vi "Create Threshold Event.vi"(0 "Threshold control":bool, 1 "Release dur. (ms)":u32, 2 "Scenario dur. (ms)":u32, 3 "Precheck dur. (ms)":u32, 5 "Threshold value":dbl, 7 "Threshold reached":bool, 9 "queue":refnum<queue>, 11 "error in":errorcluster, 13 "Queue is empty":bool) -> (15 "error out":errorcluster)   [LabVIEW 2024]
uses:
  Type Definitions/Threshold Event Parameters.ctl
  Type Definitions/Threshold Events.ctl
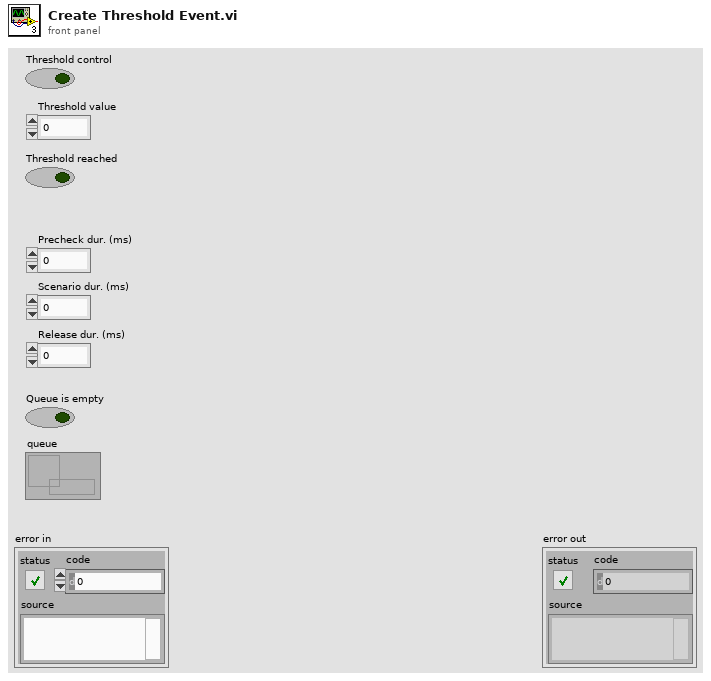
[diagram p1: front panel]
types:
  T1 = typedef "Threshold Events.ctl" = enum16{"Start Precheck", "Start Scenario", "Start Releasing", "Finish Releasing", "Clear Scenario", "Abort Scenario"}
  T2 = typedef "Threshold Event Parameters.ctl" = cluster{"Event Start time":u32, "Event name":T1, "Threshold value":dbl, "Precheck duration":u32, "Scenario Duration":u32, "Release duration":u32}
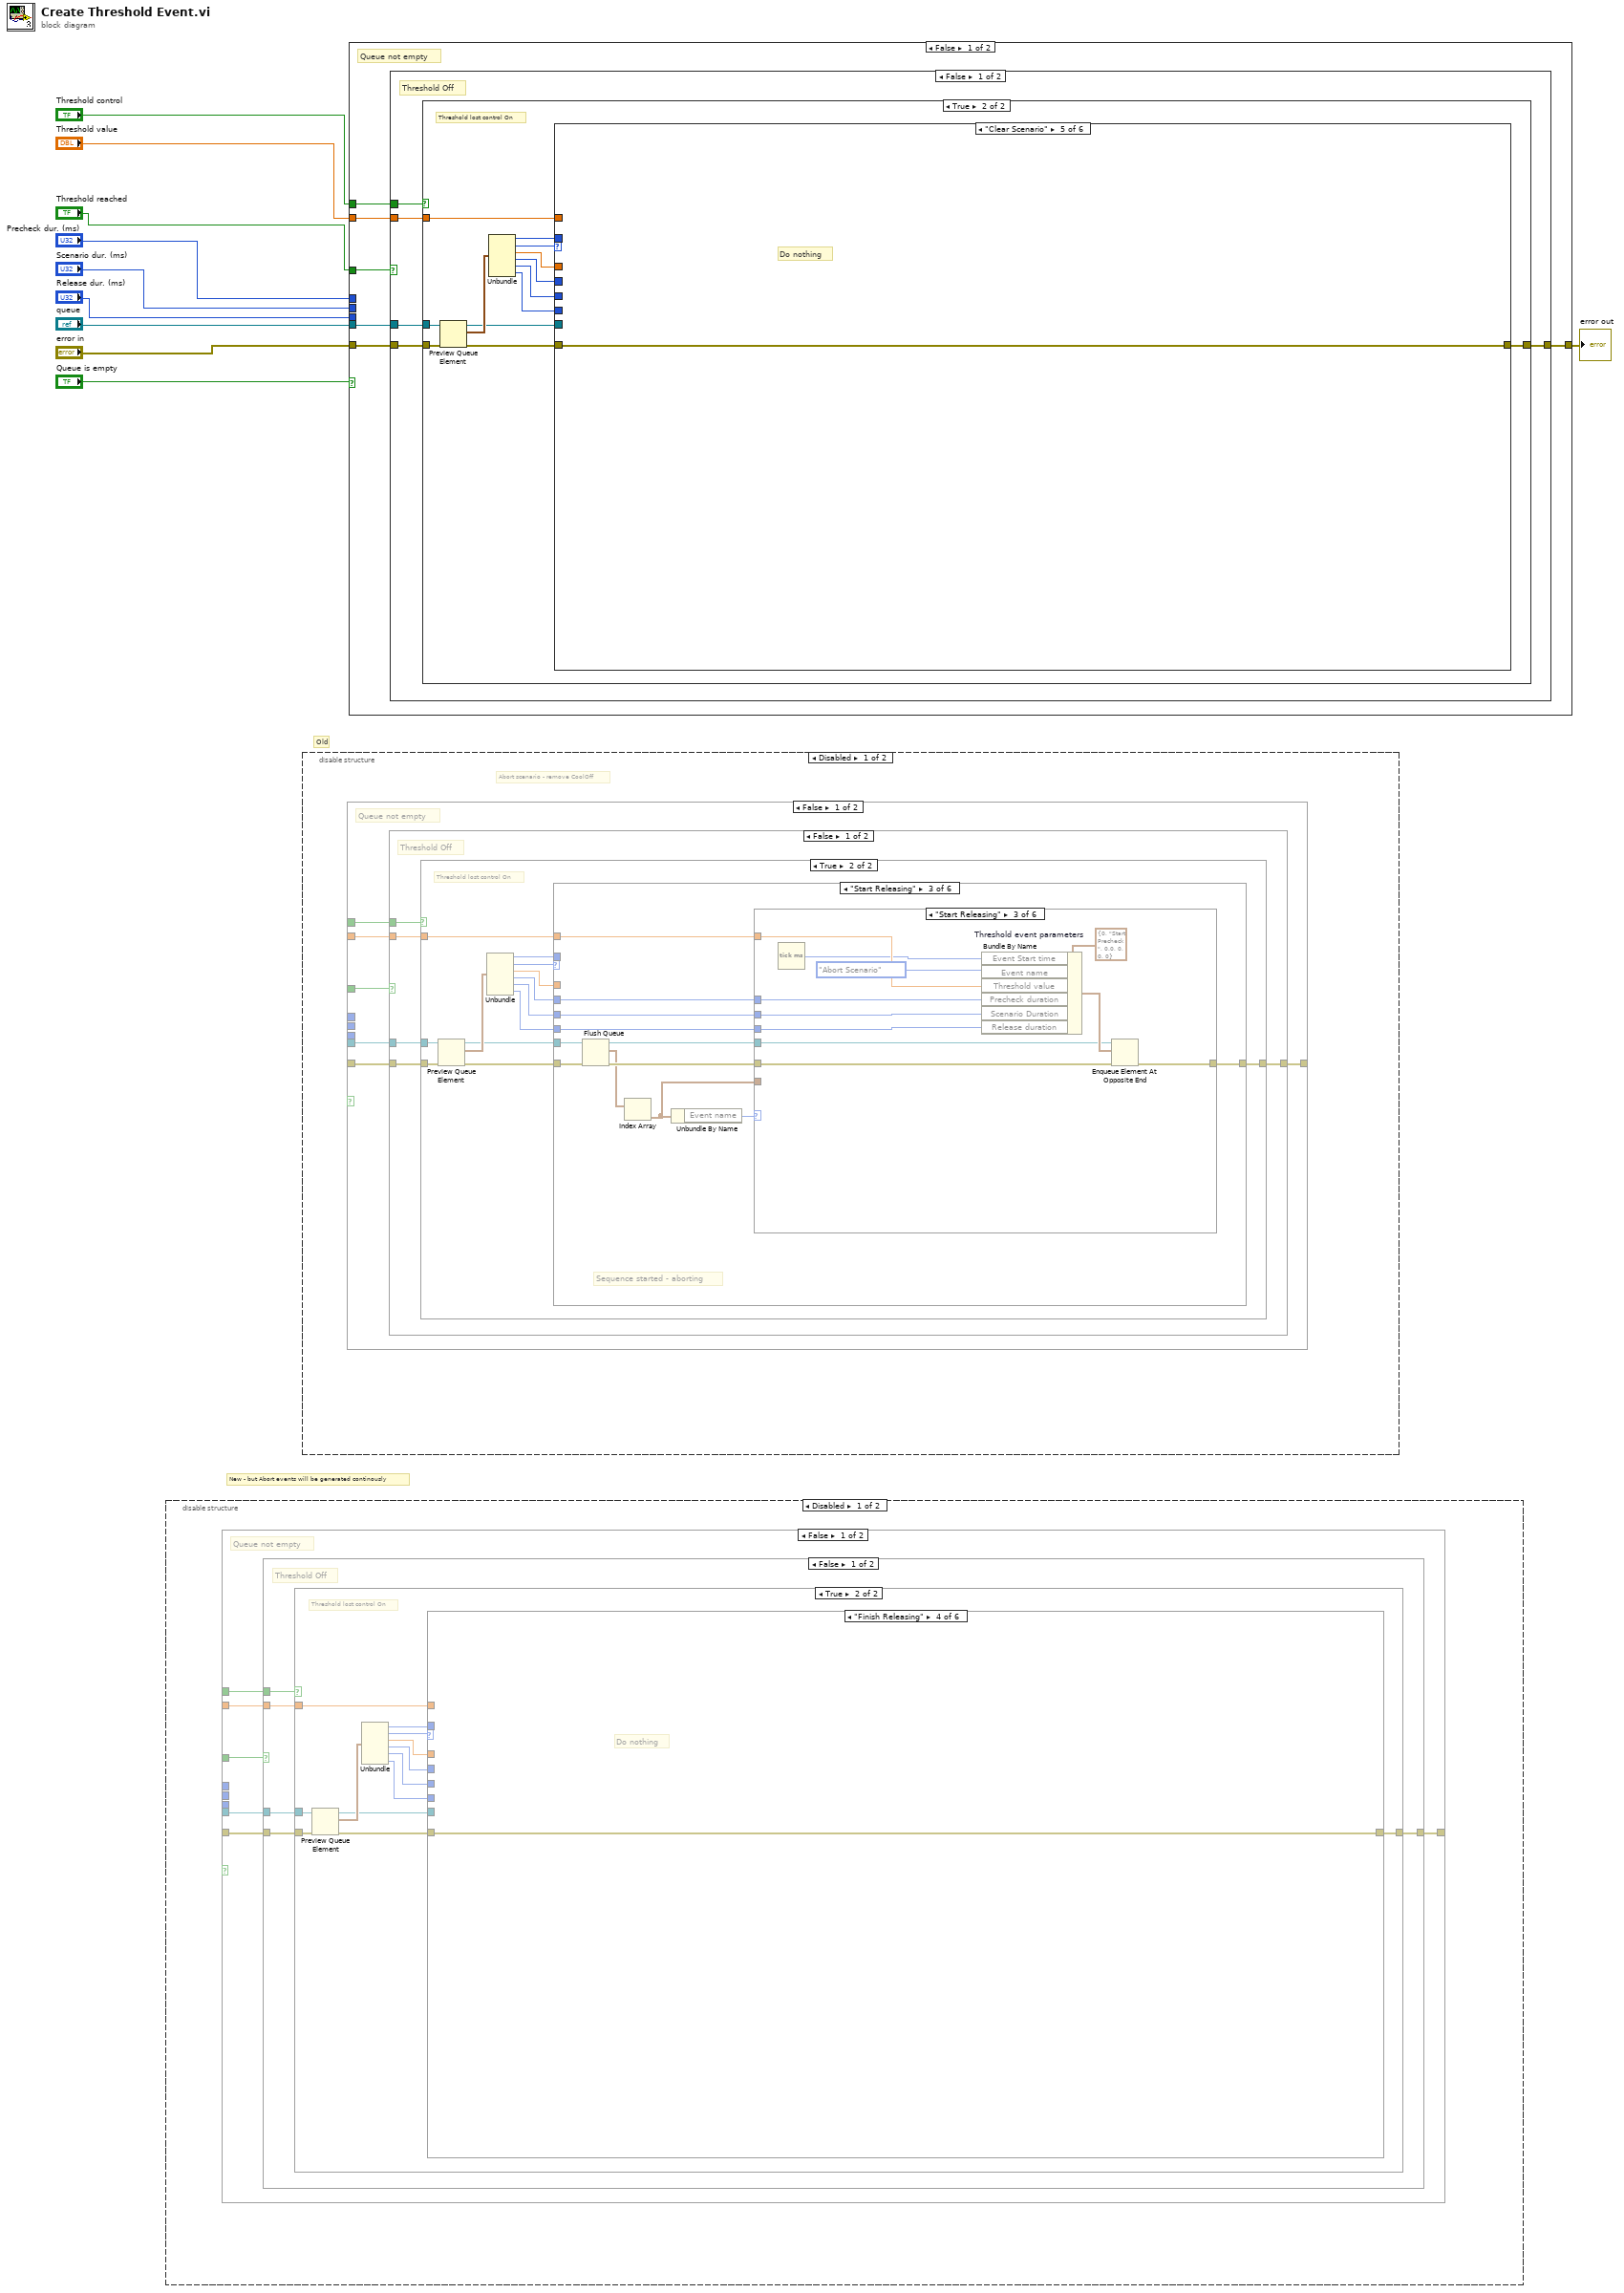
[diagram p0: block diagram]
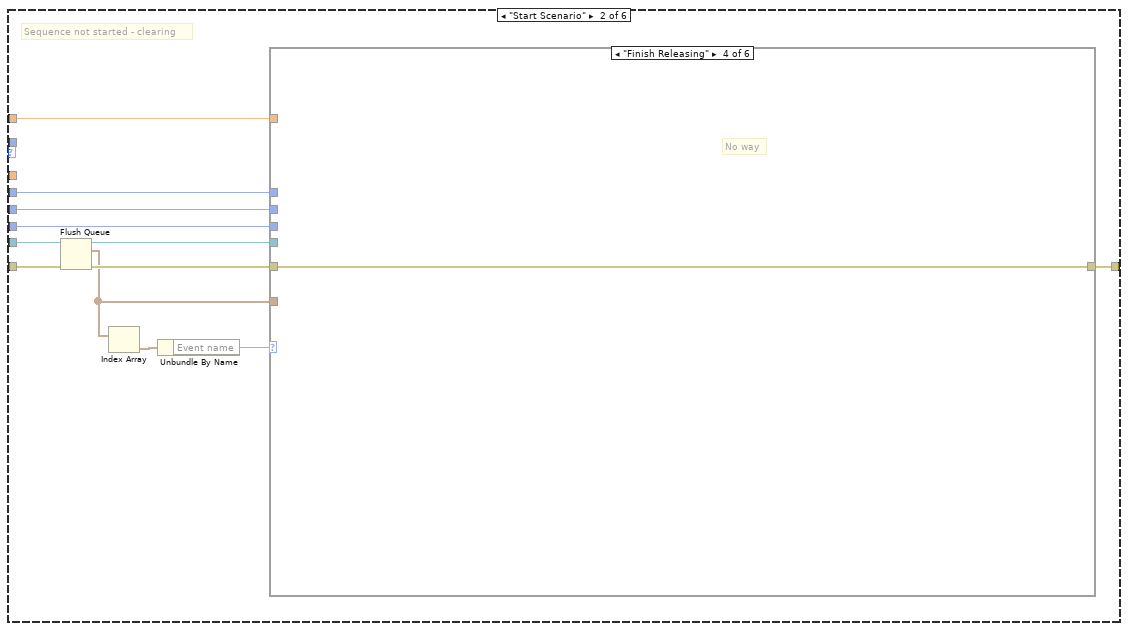
[diagram p4: hidden frame]
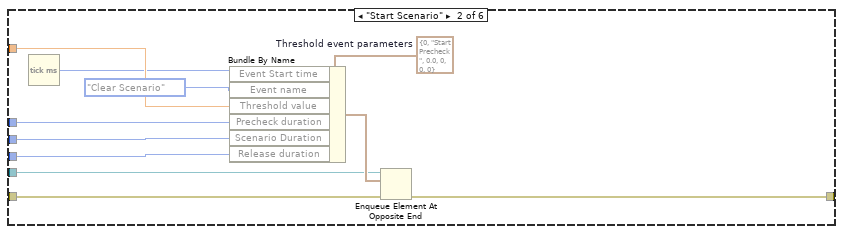
[diagram p6: hidden frame]
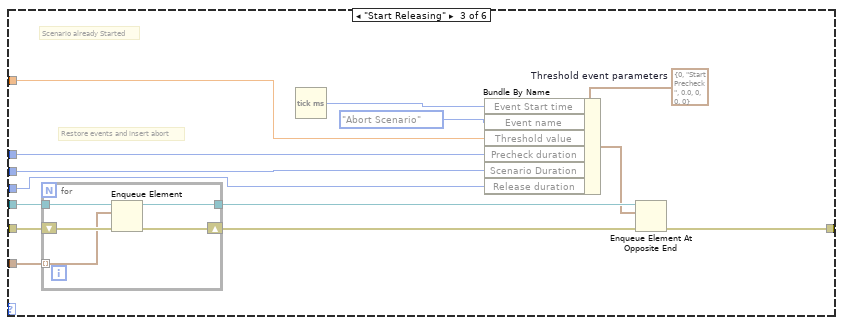
[diagram p7: hidden frame]
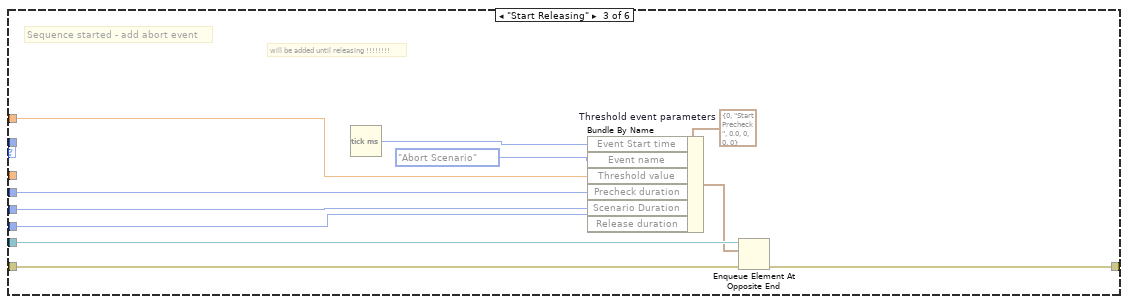
[diagram p10: hidden frame]
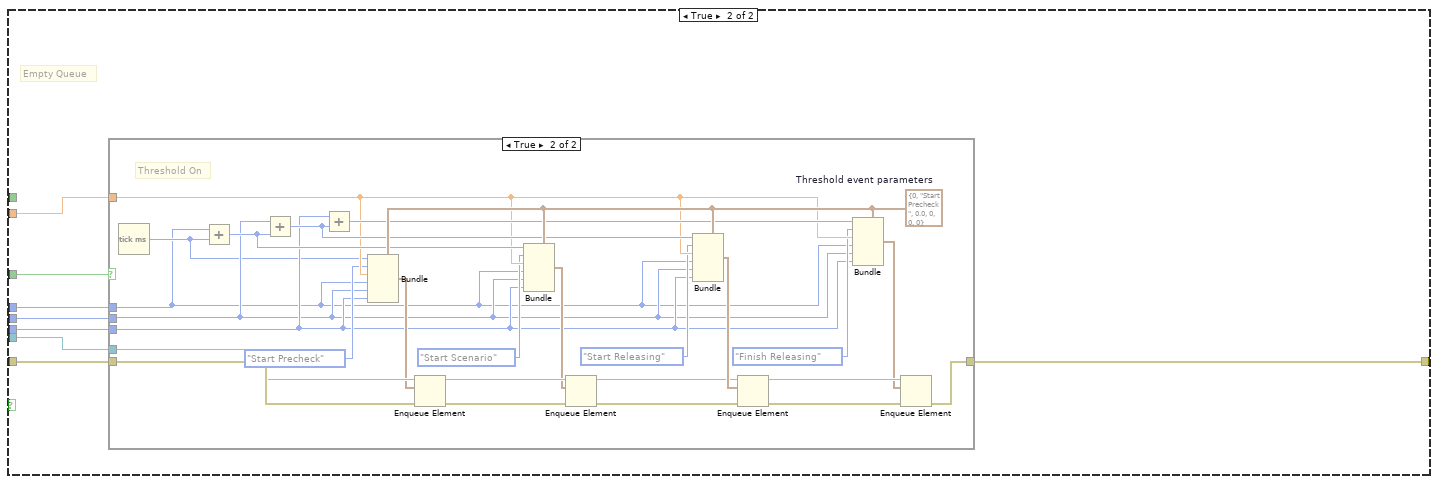
[diagram p14: hidden frame]
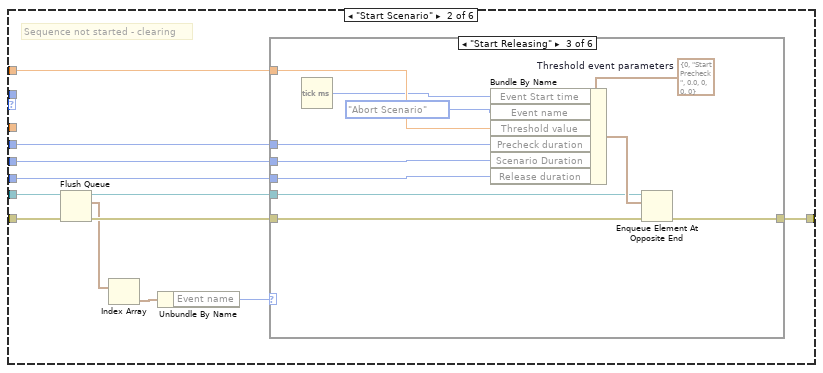
[diagram p19: hidden frame]
diagram:
  # "New - but Abort events will be generated continously"
  # "Old"
  n1 = disable-structure shown="Disabled" {
    frame Disabled {
      n2 = case shown="False" {
        selector: _ -> [_ _]
        tunnel: _ -> [w12 w105]
        tunnel: [w15 w104] -> _
        tunnel: _ -> [_ w103]
        tunnel: _ -> [_ w102]
        tunnel: _ -> [w14 w101]
        tunnel: _ -> [w16 w100]
        tunnel: _ -> [w13 w99]
        tunnel: _ -> [w11 _]
        tunnel: _ -> [_ w98]
        frame False {
          # "Queue not empty"
          n3 = case shown="False" w12 {
            tunnel: w16 -> [w21 w97]
            tunnel: [w19 w97] -> w15
            tunnel: w14 -> [w20 _]
            tunnel: w13 -> [w18 _]
            tunnel: w11 -> [w17 _]
            frame False {
              # "Threshold Off"
              n4 = case shown="True" w17 {
                tunnel: w21 -> [w22 w35]
                tunnel: w20 -> [_ w34]
                tunnel: [w22 w31] -> w19
                tunnel: w18 -> [_ w28]
                frame False {
                  # "Threshld lost control Off - skip"
                }
                frame True {
                  # "Threshold lost control On"
                  n5 = Preview Queue Element(queue=w34, error in (no error)=w35) -> (queue out=w29:refnum<queue>, element=w33:T2, error out=w32:errorcluster)  [unwired: 1 in, 1 out]
                  n6 = Unbundle(w33) -> ("Event Start time"=w27:u32, "Event name"=w30:T1, "Threshold value"=w26:dbl, "Precheck duration"=w25:u32, "Scenario Duration"=w24:u32, "Release duration"=w23:u32)
                  n7 = case shown="\"Finish Releasing\"" w30 {
                    tunnel: w32 -> [w36 w43 w88 w94 w95 w96]
                    tunnel: [w36 w48 w87 w94 w95 w96] -> w31
                    tunnel: w29 -> [_ w41 w89 _ _ _]
                    tunnel: w28 -> [_ w45 w93 _ _ _]
                    tunnel: w27 -> [_ _ _ _ _ _]
                    tunnel: w26 -> [_ _ _ _ _ _]
                    tunnel: w25 -> [_ w47 w92 _ _ _]
                    tunnel: w24 -> [_ w46 w91 _ _ _]
                    tunnel: w23 -> [_ w44 w90 _ _ _]
                    frame "Start Precheck", Default {
                      # "Do nothing"
                    }
                    frame "Start Scenario" {
                      # "Sequence not started - clearing"
                      n8 = Flush Queue(queue=w41, error in (no error)=w43) -> (queue out=w40:refnum<queue>, remaining elements=w37:T2[], error out=w42:errorcluster)
                      n9 = Index Array(array=w37) -> (element=w39:T2)  [unwired: 1 in]
                      n10 = Unbundle By Name(w39) -> ("Event name"=w38:T1)
                      n11 = case shown="\"Finish Releasing\"" w38 {
                        tunnel: [w49 w60 w70 w80 w81 w82] -> w48
                        tunnel: w47 -> [_ w56 w67 _ _ _]
                        tunnel: w46 -> [_ w55 w66 _ _ _]
                        tunnel: w45 -> [_ w54 w69 _ _ _]
                        tunnel: w44 -> [_ w53 w65 _ _ _]
                        tunnel: w42 -> [w49 w52 w74 w80 w81 w82]
                        tunnel: w40 -> [_ w51 w72 _ _ _]
                        tunnel: w37 -> [_ _ w73 _ _ _]
                        frame "Start Precheck", Default {
                          # "No way"
                        }
                        frame "Start Scenario" {
                          w59 = T2 {"Event Start time"=0, "Event name"=enum."Start Precheck", "Threshold value"=0.0, "Precheck duration"=0, "Scenario Duration"=0, "Release duration"=0}  # Threshold event parameters
                          n12 = Tick Count (ms)() -> (millisecond timer value=w50:u32)
                          n13 = Bundle By Name(cluster=w59, "Event Start time"=w50, "Event name"=Threshold_Events."Clear Scenario" ("Enum"), "Threshold value"=w54, "Precheck duration"=w56, "Scenario Duration"=w55, "Release duration"=w53) -> (w58:T2)
                          n14 = Enqueue Element At Opposite End(queue=w51, element=w58, error in (no error)=w52) -> (error out=w60:errorcluster)  [unwired: 1 in, 2 out]
                        }
                        frame "Start Releasing" {
                          w64 = T2 {"Event Start time"=0, "Event name"=enum."Start Precheck", "Threshold value"=0.0, "Precheck duration"=0, "Scenario Duration"=0, "Release duration"=0}  # Threshold event parameters
                          # "Scenario already Started"
                          # "Restore events and insert abort"
                          n15 = for {
                            shift-right: [w79] -> w71
                            shift-left: w74 -> [w78]
                            tunnel: w73 -> [w77] mode=indexing
                            tunnel: w72 -> [w76]
                            tunnel: [w75] -> w68
                            n16 = Enqueue Element(queue=w76, element=w77, error in (no error)=w78) -> (queue out=w75:refnum<queue>, error out=w79:errorcluster)  [unwired: 1 in, 1 out]
                          }
                          n17 = Tick Count (ms)() -> (millisecond timer value=w61:u32)
                          n18 = Bundle By Name(cluster=w64, "Event Start time"=w61, "Event name"=Threshold_Events."Abort Scenario" ("Enum"), "Threshold value"=w69, "Precheck duration"=w67, "Scenario Duration"=w66, "Release duration"=w65) -> (w63:T2)
                          n19 = Enqueue Element At Opposite End(queue=w68, element=w63, error in (no error)=w71) -> (error out=w70:errorcluster)  [unwired: 1 in, 2 out]
                        }
                        frame "Finish Releasing" {
                          # "No way"
                        }
                        frame "Clear Scenario" {
                          # "No way"
                        }
                        frame "Abort Scenario" {
                          # "No way"
                        }
                      }
                    }
                    frame "Start Releasing" {
                      w86 = T2 {"Event Start time"=0, "Event name"=enum."Start Precheck", "Threshold value"=0.0, "Precheck duration"=0, "Scenario Duration"=0, "Release duration"=0}  # Threshold event parameters
                      # "will be added until releasing !!!!!!!!"
                      # "Sequence started - add abort event"
                      n20 = Tick Count (ms)() -> (millisecond timer value=w83:u32)
                      n21 = Bundle By Name(cluster=w86, "Event Start time"=w83, "Event name"=Threshold_Events."Abort Scenario" ("Enum"), "Threshold value"=w93, "Precheck duration"=w92, "Scenario Duration"=w91, "Release duration"=w90) -> (w85:T2)
                      n22 = Enqueue Element At Opposite End(queue=w89, element=w85, error in (no error)=w88) -> (error out=w87:errorcluster)  [unwired: 1 in, 2 out]
                    }
                    frame "Finish Releasing" {
                      # "Do nothing"
                    }
                    frame "Clear Scenario" {
                      # "Do nothing"
                    }
                    frame "Abort Scenario" {
                      # "Do nothing"
                    }
                  }
                }
              }
            }
            frame True {
              # "Threshold On - Skip"
            }
          }
        }
        frame True {
          # "Empty Queue"
          n23 = case shown="True" w105 {
            tunnel: w103 -> [_ w109]
            tunnel: w100 -> [w106 w132]
            tunnel: [w106 w126] -> w104
            tunnel: w101 -> [_ w131]
            tunnel: w102 -> [_ w110]
            tunnel: w99 -> [_ w116]
            tunnel: w98 -> [_ w107]
            frame False {
              # "Threshold Off"
            }
            frame True {
              w121 = T2 {"Event Start time"=0, "Event name"=enum."Start Precheck", "Threshold value"=0.0, "Precheck duration"=0, "Scenario Duration"=0, "Release duration"=0}  # Threshold event parameters
              # "Threshold On"
              n24 = Tick Count (ms)() -> (millisecond timer value=w108:u32)
              n25 = Add(x=w107, y=w108) -> (x+y=w119:u32)
              n26 = Add(x=w109, y=w119) -> (x+y=w117:u32)
              n27 = Add(x=w110, y=w117) -> (x+y=w118:u32)
              n28 = Bundle(cluster=w121, "Event Start time"=w108, "Event name"=Threshold_Events."Start Precheck" ("Enum"), "Threshold value"=w116, "Precheck duration"=w107, "Scenario Duration"=w109, "Release duration"=w110) -> (w120:T2)
              n29 = Enqueue Element(queue=w131, element=w120, error in (no error)=w132) -> (queue out=w129:refnum<queue>, error out=w130:errorcluster)  [unwired: 1 in, 1 out]
              n30 = Bundle(cluster=w121, "Event Start time"=w119, "Event name"=Threshold_Events."Start Scenario" ("Enum"), "Threshold value"=w116, "Precheck duration"=w107, "Scenario Duration"=w109, "Release duration"=w110) -> (w113:T2)
              n31 = Enqueue Element(queue=w129, element=w113, error in (no error)=w130) -> (queue out=w124:refnum<queue>, error out=w128:errorcluster)  [unwired: 1 in, 1 out]
              n32 = Bundle(cluster=w121, "Event Start time"=w117, "Event name"=Threshold_Events."Start Releasing" ("Enum"), "Threshold value"=w116, "Precheck duration"=w107, "Scenario Duration"=w109, "Release duration"=w110) -> (w125:T2)
              n33 = Enqueue Element(queue=w124, element=w125, error in (no error)=w128) -> (queue out=w123:refnum<queue>, error out=w127:errorcluster)  [unwired: 1 in, 1 out]
              n34 = Bundle(cluster=w121, "Event Start time"=w118, "Event name"=Threshold_Events."Finish Releasing" ("Enum"), "Threshold value"=w116, "Precheck duration"=w107, "Scenario Duration"=w109, "Release duration"=w110) -> (w122:T2)
              n35 = Enqueue Element(queue=w123, element=w122, error in (no error)=w127) -> (error out=w126:errorcluster)  [unwired: 1 in, 2 out]
            }
          }
        }
      }
    }
    frame Enabled {
    }
  }
  n36 = disable-structure shown="Disabled" {
    frame Disabled {
      # "Abort scenario - remove CoolOff"
      n37 = case shown="False" {
        selector: _ -> [_ _]
        tunnel: _ -> [w134 w239]
        tunnel: [w137 w238] -> _
        tunnel: _ -> [_ w237]
        tunnel: _ -> [_ w236]
        tunnel: _ -> [w136 w235]
        tunnel: _ -> [w138 w234]
        tunnel: _ -> [w135 w233]
        tunnel: _ -> [w133 _]
        tunnel: _ -> [_ w232]
        frame False {
          # "Queue not empty"
          n38 = case shown="False" w134 {
            tunnel: w138 -> [w143 w231]
            tunnel: [w141 w231] -> w137
            tunnel: w136 -> [w142 _]
            tunnel: w135 -> [w140 _]
            tunnel: w133 -> [w139 _]
            frame False {
              # "Threshold Off"
              n39 = case shown="True" w139 {
                tunnel: w143 -> [w144 w157]
                tunnel: w142 -> [_ w156]
                tunnel: [w144 w153] -> w141
                tunnel: w140 -> [_ w150]
                frame False {
                  # "Threshld lost control Off - skip"
                }
                frame True {
                  # "Threshold lost control On"
                  n40 = Preview Queue Element(queue=w156, error in (no error)=w157) -> (queue out=w151:refnum<queue>, element=w155:T2, error out=w154:errorcluster)  [unwired: 1 in, 1 out]
                  n41 = Unbundle(w155) -> ("Event Start time"=w149:u32, "Event name"=w152:T1, "Threshold value"=w148:dbl, "Precheck duration"=w147:u32, "Scenario Duration"=w146:u32, "Release duration"=w145:u32)
                  n42 = case shown="\"Start Releasing\"" w152 {
                    tunnel: w154 -> [w158 w165 w203 w228 w229 w230]
                    tunnel: [w158 w170 w208 w228 w229 w230] -> w153
                    tunnel: w151 -> [_ w163 w201 _ _ _]
                    tunnel: w150 -> [_ w167 w205 _ _ _]
                    tunnel: w149 -> [_ _ _ _ _ _]
                    tunnel: w148 -> [_ _ _ _ _ _]
                    tunnel: w147 -> [_ w169 w207 _ _ _]
                    tunnel: w146 -> [_ w168 w206 _ _ _]
                    tunnel: w145 -> [_ w166 w204 _ _ _]
                    frame "Start Precheck", Default {
                      # "Do nothing"
                    }
                    frame "Start Scenario" {
                      # "Sequence not started - clearing"
                      n43 = Flush Queue(queue=w163, error in (no error)=w165) -> (queue out=w162:refnum<queue>, remaining elements=w161:T2[], error out=w164:errorcluster)
                      n44 = Index Array(array=w161) -> (element=w160:T2)  [unwired: 1 in]
                      n45 = Unbundle By Name(w160) -> ("Event name"=w159:T1)
                      n46 = case shown="\"Start Releasing\"" w159 {
                        tunnel: [w171 w182 w193 w194 w195 w196] -> w170
                        tunnel: w169 -> [_ w178 w189 _ _ _]
                        tunnel: w168 -> [_ w177 w188 _ _ _]
                        tunnel: w167 -> [_ w176 w187 _ _ _]
                        tunnel: w166 -> [_ w175 w186 _ _ _]
                        tunnel: w164 -> [w171 w174 w185 w194 w195 w196]
                        tunnel: w162 -> [_ w173 w184 _ _ _]
                        frame "Start Precheck", Default {
                          # "No way"
                        }
                        frame "Start Scenario" {
                          w181 = T2 {"Event Start time"=0, "Event name"=enum."Start Precheck", "Threshold value"=0.0, "Precheck duration"=0, "Scenario Duration"=0, "Release duration"=0}  # Threshold event parameters
                          n47 = Tick Count (ms)() -> (millisecond timer value=w172:u32)
                          n48 = Bundle By Name(cluster=w181, "Event Start time"=w172, "Event name"=Threshold_Events."Clear Scenario" ("Enum"), "Threshold value"=w176, "Precheck duration"=w178, "Scenario Duration"=w177, "Release duration"=w175) -> (w180:T2)
                          n49 = Enqueue Element At Opposite End(queue=w173, element=w180, error in (no error)=w174) -> (error out=w182:errorcluster)  [unwired: 1 in, 2 out]
                        }
                        frame "Start Releasing" {
                          w192 = T2 {"Event Start time"=0, "Event name"=enum."Start Precheck", "Threshold value"=0.0, "Precheck duration"=0, "Scenario Duration"=0, "Release duration"=0}  # Threshold event parameters
                          n50 = Tick Count (ms)() -> (millisecond timer value=w183:u32)
                          n51 = Bundle By Name(cluster=w192, "Event Start time"=w183, "Event name"=Threshold_Events."Abort Scenario" ("Enum"), "Threshold value"=w187, "Precheck duration"=w189, "Scenario Duration"=w188, "Release duration"=w186) -> (w191:T2)
                          n52 = Enqueue Element At Opposite End(queue=w184, element=w191, error in (no error)=w185) -> (error out=w193:errorcluster)  [unwired: 1 in, 2 out]
                        }
                        frame "Finish Releasing" {
                          # "No way"
                        }
                        frame "Clear Scenario" {
                          # "No way"
                        }
                        frame "Abort Scenario" {
                          # "No way"
                        }
                      }
                    }
                    frame "Start Releasing" {
                      # "Sequence started - aborting"
                      n53 = Flush Queue(queue=w201, error in (no error)=w203) -> (queue out=w200:refnum<queue>, remaining elements=w199:T2[], error out=w202:errorcluster)
                      n54 = Index Array(array=w199) -> (element=w197:T2)  [unwired: 1 in]
                      n55 = Unbundle By Name(w197) -> ("Event name"=w198:T1)
                      n56 = case shown="\"Start Releasing\"" w198 {
                        tunnel: [w209 w210 w221 w224 w226 w227] -> w208
                        tunnel: w207 -> [_ _ w217 _ _ _]
                        tunnel: w206 -> [_ _ w216 _ _ _]
                        tunnel: w205 -> [_ _ w215 _ _ _]
                        tunnel: w204 -> [_ _ w214 _ _ _]
                        tunnel: w202 -> [w209 w210 w212 w225 w226 w227]
                        tunnel: w200 -> [_ _ w211 w222 _ _]
                        tunnel: w197 -> [_ _ _ w223 _ _]
                        frame "Start Precheck", Default {
                          # "No way"
                        }
                        frame "Start Scenario" {
                          # "No Way"
                        }
                        frame "Start Releasing" {
                          w220 = T2 {"Event Start time"=0, "Event name"=enum."Start Precheck", "Threshold value"=0.0, "Precheck duration"=0, "Scenario Duration"=0, "Release duration"=0}  # Threshold event parameters
                          n57 = Tick Count (ms)() -> (millisecond timer value=w213:u32)
                          n58 = Bundle By Name(cluster=w220, "Event Start time"=w213, "Event name"=Threshold_Events."Abort Scenario" ("Enum"), "Threshold value"=w215, "Precheck duration"=w217, "Scenario Duration"=w216, "Release duration"=w214) -> (w219:T2)
                          n59 = Enqueue Element At Opposite End(queue=w211, element=w219, error in (no error)=w212) -> (error out=w221:errorcluster)  [unwired: 1 in, 2 out]
                        }
                        frame "Finish Releasing" {
                          # "Restore Finish Releasing"
                          n60 = Enqueue Element(queue=w222, element=w223, error in (no error)=w225) -> (error out=w224:errorcluster)  [unwired: 1 in, 2 out]
                        }
                        frame "Clear Scenario" {
                          # "No Way"
                        }
                        frame "Abort Scenario" {
                          # "No Way"
                        }
                      }
                    }
                    frame "Finish Releasing" {
                      # "Do nothing"
                    }
                    frame "Clear Scenario" {
                      # "Do nothing"
                    }
                    frame "Abort Scenario" {
                      # "Do nothing"
                    }
                  }
                }
              }
            }
            frame True {
              # "Threshold On - Skip"
            }
          }
        }
        frame True {
          # "Empty Queue"
          n61 = case shown="False" w239 {
            tunnel: w237 -> [_ w243]
            tunnel: w234 -> [w240 w266]
            tunnel: [w240 w260] -> w238
            tunnel: w235 -> [_ w265]
            tunnel: w236 -> [_ w244]
            tunnel: w233 -> [_ w250]
            tunnel: w232 -> [_ w241]
            frame False {
              # "Threshold Off"
            }
            frame True {
              w255 = T2 {"Event Start time"=0, "Event name"=enum."Start Precheck", "Threshold value"=0.0, "Precheck duration"=0, "Scenario Duration"=0, "Release duration"=0}  # Threshold event parameters
              # "Threshold On"
              n62 = Tick Count (ms)() -> (millisecond timer value=w242:u32)
              n63 = Add(x=w241, y=w242) -> (x+y=w253:u32)
              n64 = Add(x=w243, y=w253) -> (x+y=w251:u32)
              n65 = Add(x=w244, y=w251) -> (x+y=w252:u32)
              n66 = Bundle(cluster=w255, "Event Start time"=w242, "Event name"=Threshold_Events."Start Precheck" ("Enum"), "Threshold value"=w250, "Precheck duration"=w241, "Scenario Duration"=w243, "Release duration"=w244) -> (w254:T2)
              n67 = Enqueue Element(queue=w265, element=w254, error in (no error)=w266) -> (queue out=w263:refnum<queue>, error out=w264:errorcluster)  [unwired: 1 in, 1 out]
              n68 = Bundle(cluster=w255, "Event Start time"=w253, "Event name"=Threshold_Events."Start Scenario" ("Enum"), "Threshold value"=w250, "Precheck duration"=w241, "Scenario Duration"=w243, "Release duration"=w244) -> (w247:T2)
              n69 = Enqueue Element(queue=w263, element=w247, error in (no error)=w264) -> (queue out=w258:refnum<queue>, error out=w262:errorcluster)  [unwired: 1 in, 1 out]
              n70 = Bundle(cluster=w255, "Event Start time"=w251, "Event name"=Threshold_Events."Start Releasing" ("Enum"), "Threshold value"=w250, "Precheck duration"=w241, "Scenario Duration"=w243, "Release duration"=w244) -> (w259:T2)
              n71 = Enqueue Element(queue=w258, element=w259, error in (no error)=w262) -> (queue out=w257:refnum<queue>, error out=w261:errorcluster)  [unwired: 1 in, 1 out]
              n72 = Bundle(cluster=w255, "Event Start time"=w252, "Event name"=Threshold_Events."Finish Releasing" ("Enum"), "Threshold value"=w250, "Precheck duration"=w241, "Scenario Duration"=w243, "Release duration"=w244) -> (w256:T2)
              n73 = Enqueue Element(queue=w257, element=w256, error in (no error)=w261) -> (error out=w260:errorcluster)  [unwired: 1 in, 2 out]
            }
          }
        }
      }
    }
    frame Enabled {
    }
  }
  n74 = case shown="False" "Queue is empty" {
    tunnel: "Threshold reached" -> [w268 w341]
    tunnel: [w271 w340] -> w10
    tunnel: "Scenario dur. (ms)" -> [_ w339]
    tunnel: "Release dur. (ms)" -> [_ w338]
    tunnel: "queue" -> [w270 w337]
    tunnel: "error in" -> [w272 w336]
    tunnel: "Threshold value" -> [w269 w335]
    tunnel: "Threshold control" -> [w267 _]
    tunnel: "Precheck dur. (ms)" -> [_ w334]
    frame False {
      # "Queue not empty"
      n75 = case shown="False" w268 {
        tunnel: w272 -> [w277 w333]
        tunnel: [w275 w333] -> w271
        tunnel: w270 -> [w276 _]
        tunnel: w269 -> [w274 _]
        tunnel: w267 -> [w273 _]
        frame False {
          # "Threshold Off"
          n76 = case shown="True" w273 {
            tunnel: w277 -> [w278 w291]
            tunnel: w276 -> [_ w290]
            tunnel: [w278 w287] -> w275
            tunnel: w274 -> [_ w284]
            frame False {
              # "Threshld lost control Off - skip"
            }
            frame True {
              # "Threshold lost control On"
              n77 = Preview Queue Element(queue=w290, error in (no error)=w291) -> (queue out=w285:refnum<queue>, element=w289:T2, error out=w288:errorcluster)  [unwired: 1 in, 1 out]
              n78 = Unbundle(w289) -> ("Event Start time"=w283:u32, "Event name"=w286:T1, "Threshold value"=w282:dbl, "Precheck duration"=w281:u32, "Scenario Duration"=w280:u32, "Release duration"=w279:u32)
              n79 = case shown="\"Clear Scenario\"" w286 {
                tunnel: w288 -> [w292 w299 w329 w330 w331 w332]
                tunnel: [w292 w304 w329 w330 w331 w332] -> w287
                tunnel: w285 -> [_ w297 _ _ _ _]
                tunnel: w284 -> [_ w301 _ _ _ _]
                tunnel: w283 -> [_ _ _ _ _ _]
                tunnel: w282 -> [_ _ _ _ _ _]
                tunnel: w281 -> [_ w303 _ _ _ _]
                tunnel: w280 -> [_ w302 _ _ _ _]
                tunnel: w279 -> [_ w300 _ _ _ _]
                frame "Start Precheck", Default {
                  # "Do nothing"
                }
                frame "Start Scenario" {
                  # "Sequence not started - clearing"
                  n80 = Flush Queue(queue=w297, error in (no error)=w299) -> (queue out=w296:refnum<queue>, remaining elements=w293:T2[], error out=w298:errorcluster)
                  n81 = Index Array(array=w293) -> (element=w295:T2)  [unwired: 1 in]
                  n82 = Unbundle By Name(w295) -> ("Event name"=w294:T1)
                  n83 = case shown="\"Finish Releasing\"" w294 {
                    tunnel: [w305 w316 w317 w326 w327 w328] -> w304
                    tunnel: w303 -> [_ w312 _ _ _ _]
                    tunnel: w302 -> [_ w311 _ _ _ _]
                    tunnel: w301 -> [_ w310 _ _ _ _]
                    tunnel: w300 -> [_ w309 _ _ _ _]
                    tunnel: w298 -> [w305 w308 w320 w326 w327 w328]
                    tunnel: w296 -> [_ w307 w318 _ _ _]
                    tunnel: w293 -> [_ _ w319 _ _ _]
                    frame "Start Precheck", Default {
                      # "No way"
                    }
                    frame "Start Scenario" {
                      w315 = T2 {"Event Start time"=0, "Event name"=enum."Start Precheck", "Threshold value"=0.0, "Precheck duration"=0, "Scenario Duration"=0, "Release duration"=0}  # Threshold event parameters
                      n84 = Tick Count (ms)() -> (millisecond timer value=w306:u32)
                      n85 = Bundle By Name(cluster=w315, "Event Start time"=w306, "Event name"=Threshold_Events."Clear Scenario" ("Enum"), "Threshold value"=w310, "Precheck duration"=w312, "Scenario Duration"=w311, "Release duration"=w309) -> (w314:T2)
                      n86 = Enqueue Element At Opposite End(queue=w307, element=w314, error in (no error)=w308) -> (error out=w316:errorcluster)  [unwired: 1 in, 2 out]
                    }
                    frame "Start Releasing" {
                      # "Scenario already Started"
                      # "Restore events"
                      n87 = for {
                        shift-right: [w325] -> w317
                        shift-left: w320 -> [w324]
                        tunnel: w319 -> [w323] mode=indexing
                        tunnel: w318 -> [w322]
                        tunnel: [w321] -> _
                        n88 = Enqueue Element(queue=w322, element=w323, error in (no error)=w324) -> (queue out=w321:refnum<queue>, error out=w325:errorcluster)  [unwired: 1 in, 1 out]
                      }
                    }
                    frame "Finish Releasing" {
                      # "No way"
                    }
                    frame "Clear Scenario" {
                      # "No way"
                    }
                    frame "Abort Scenario" {
                      # "No way"
                    }
                  }
                }
                frame "Start Releasing" {
                  # "Sequence started - do nothing"
                }
                frame "Finish Releasing" {
                  # "Do nothing"
                }
                frame "Clear Scenario" {
                  # "Do nothing"
                }
                frame "Abort Scenario" {
                  # "Do nothing"
                }
              }
            }
          }
        }
        frame True {
          # "Threshold On - Skip"
        }
      }
    }
    frame True {
      # "Empty Queue"
      n89 = case shown="True" w341 {
        tunnel: w339 -> [_ w345]
        tunnel: w336 -> [w342 w368]
        tunnel: [w342 w362] -> w340
        tunnel: w337 -> [_ w367]
        tunnel: w338 -> [_ w346]
        tunnel: w335 -> [_ w352]
        tunnel: w334 -> [_ w343]
        frame False {
          # "Threshold Off"
        }
        frame True {
          w357 = T2 {"Event Start time"=0, "Event name"=enum."Start Precheck", "Threshold value"=0.0, "Precheck duration"=0, "Scenario Duration"=0, "Release duration"=0}  # Threshold event parameters
          # "Threshold On"
          n90 = Tick Count (ms)() -> (millisecond timer value=w344:u32)
          n91 = Add(x=w343, y=w344) -> (x+y=w355:u32)
          n92 = Add(x=w345, y=w355) -> (x+y=w353:u32)
          n93 = Add(x=w346, y=w353) -> (x+y=w354:u32)
          n94 = Bundle(cluster=w357, "Event Start time"=w344, "Event name"=Threshold_Events."Start Precheck" ("Enum"), "Threshold value"=w352, "Precheck duration"=w343, "Scenario Duration"=w345, "Release duration"=w346) -> (w356:T2)
          n95 = Enqueue Element(queue=w367, element=w356, error in (no error)=w368) -> (queue out=w365:refnum<queue>, error out=w366:errorcluster)  [unwired: 1 in, 1 out]
          n96 = Bundle(cluster=w357, "Event Start time"=w355, "Event name"=Threshold_Events."Start Scenario" ("Enum"), "Threshold value"=w352, "Precheck duration"=w343, "Scenario Duration"=w345, "Release duration"=w346) -> (w349:T2)
          n97 = Enqueue Element(queue=w365, element=w349, error in (no error)=w366) -> (queue out=w360:refnum<queue>, error out=w364:errorcluster)  [unwired: 1 in, 1 out]
          n98 = Bundle(cluster=w357, "Event Start time"=w353, "Event name"=Threshold_Events."Start Releasing" ("Enum"), "Threshold value"=w352, "Precheck duration"=w343, "Scenario Duration"=w345, "Release duration"=w346) -> (w361:T2)
          n99 = Enqueue Element(queue=w360, element=w361, error in (no error)=w364) -> (queue out=w359:refnum<queue>, error out=w363:errorcluster)  [unwired: 1 in, 1 out]
          n100 = Bundle(cluster=w357, "Event Start time"=w354, "Event name"=Threshold_Events."Finish Releasing" ("Enum"), "Threshold value"=w352, "Precheck duration"=w343, "Scenario Duration"=w345, "Release duration"=w346) -> (w358:T2)
          n101 = Enqueue Element(queue=w359, element=w358, error in (no error)=w363) -> (error out=w362:errorcluster)  [unwired: 1 in, 2 out]
        }
      }
    }
  }
  "error out" <- w10
